vi "Aplicacion.vi"() -> ()   [LabVIEW 2016]
uses:
  <vilib>/addons/database/Connection.llb/Conn ObjectReference.ctl
  <vilib>/addons/database/Connection.llb/DB Tools Open Connec (Path).vi
  <vilib>/Instr/_visa.llb/VISA Configure Serial Port (Instr).vi
  <vilib>/addons/database/Connection.llb/Conn Execute.vi
  <vilib>/addons/database/Recordset.llb/Rec Destroy - Connection.vi
  <vilib>/Utility/config.llb/Read Key (String).vi
  <vilib>/Utility/config.llb/Write Key (String).vi
  <vilib>/addons/database/NI_Database_API.lvlib
  <vilib>/Utility/config.llb/NI_LVConfig.lvlib
panel:
  out "Ready":bool
  out "Condition":string
  out "Table":string
  in  "Read/Write Auto":bool
  out "retry":bool=TRUE
  out "Errores":errorcluster[](array[cluster])
  in  "Retry Conection":bool
  out "Errors":string[](array[string])
  in  "Configuration":bool caption="Blank Button"
  in  "Registers":bool caption="Blank Button"
  in  "Monitor":bool caption="Blank Button"
  in  "Tab Control":enum32{"Monitor", "Registers", "Configuration"}(tab)
  out "Graph":dbl(graph)
  in  "Conection Type":string(combo)="VISA"
  in  "To":timestamp
  in  "From":timestamp
  out "Data":i32(listbox)
  in  "Get Data":bool
  in  "Aply filter":bool
  in  "Section":string(combo)
  in  "Edit Config":bool
  in  "Data":string[][](table)
  in  "Save":bool
  in  "Delete Data":bool
  out "Modbus Request":string
  in  "Quantity":u8=1
  in  "Address":u8=1
  in  "Function Code":u8(ring)=1 items=["Read Coils"=1, "Read Discrete Inputs"=2, "Read Holding Registers"=3, "Read Input Register"=4, "Write Single Coil"=5, "Write Single Register"=6]
  out "Conections":T1
  out "Byte Count":i32 format="%02.0f"
  out "Function Code":i32 format="%02.0f"
  in  "Conection":string(combo)="VISA"
  in  "Read/Write Data":bool
  out "Modbus Response":string
  out "Data":dbl format="%#_4g"
  in  "parity (0:none)":enum16{"None", "Odd", "Even", "Mark", "Space"}(ring)
  in  "Cluster Conections":T1 {"VISAs"."Stop bit" items=["1.0"=10, "1.5"=15, "2.0"=20]; "VISAs"."Parity" items=["No parity", "Odd parity", "Even parity", "Mark parity", "Space parity"]}
  out "Final Error":errorcluster
  in  "stop":bool
  # "Universidad Autonoma de Queretaro"
  # "Facultad de Informatica"
  # "Desarrollo de Intefaces de Hardware II"
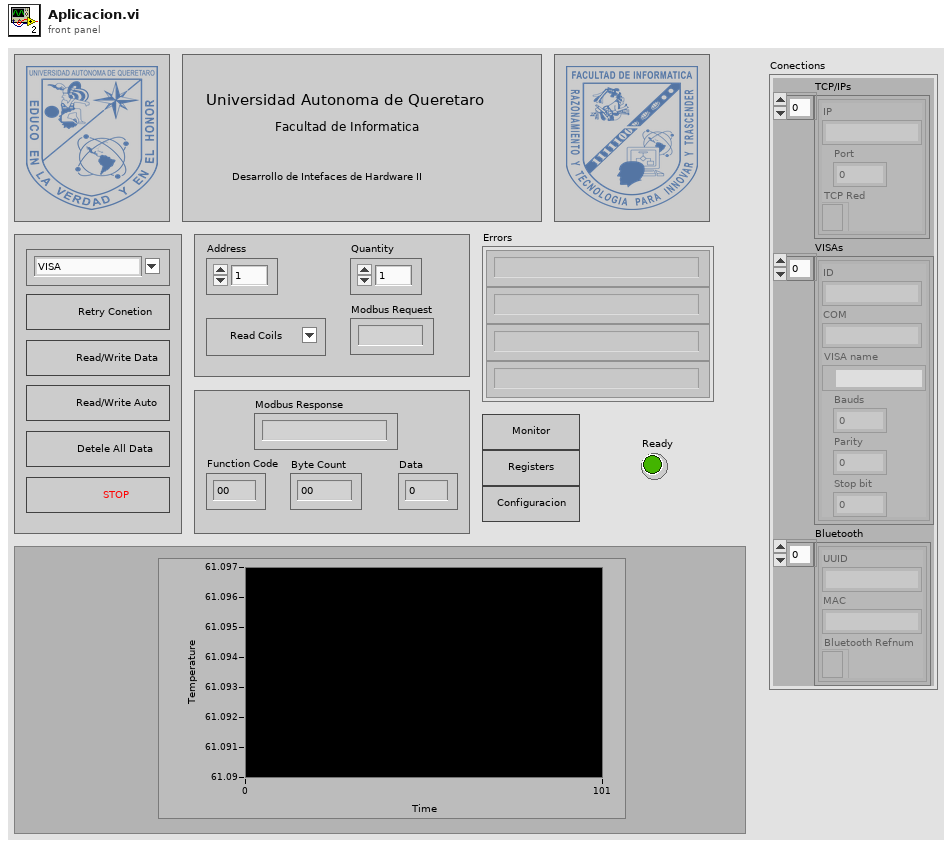
[diagram p1: front panel]
types:
  T1 = cluster{"TCP/IPs":cluster{"IP":string, "Port":u16, "TCP Red":refnum<k5>}[], "VISAs":cluster{"ID":string, "COM":string, "VISA name":refnum<visa-resource-name>, "Bauds":dbl, "Parity":u16, "Stop bit":u16}[], "Bluetooth":cluster{"UUID":string, "MAC":string, "Bluetooth Refnum":refnum<k31>}[]}
  T2 = enum16{"Standard", "Buffered", "CRLF", "Immediate"}
  T3 = enum8{"Enabled", "Disabled", "Disabled and Grayed Out"}
  T4 = typedef "NI_LVConfig.lvlib/Config Data RefNum.ctl" = refnum<k1>
  T5 = typedef "NI_Database_API.lvlib/Conn ObjectReference.ctl" = refnum<k1>
  T6 = cluster{"IP":string, "Port":u16, "TCP Red":refnum<k5>}[]
  T7 = cluster{"IP":string, "Port":u16, "TCP Red":refnum<k5>}
  T8 = cluster{"IP":string, "Port":u16, "connection ID":refnum<k5>}
  T9 = cluster{"IP":string, "Port":u16, "connection ID":refnum<k5>}[]
  T10 = cluster{"ID":string, "COM":string, "VISA name":refnum<visa-resource-name>, "Bauds":dbl, "Parity":u16, "Stop bit":u16}[]
  T11 = cluster{"ID":string, "COM":string, "VISA name":refnum<visa-resource-name>, "Bauds":dbl, "Parity":u16, "Stop bit":u16}
  T12 = cluster{"UUID":string, "MAC":string, "Bluetooth Refnum":refnum<k31>}[]
  T13 = cluster{"UUID":string, "MAC":string, "Bluetooth Refnum":refnum<k31>}
  T14 = cluster{"UUID":string, "UUID":string, "connection ID":refnum<k31>}
  T15 = cluster{"UUID":string, "UUID":string, "connection ID":refnum<k31>}[]
  T16 = typedef "NI_Database_API.lvlib/Rec ObjectReference.ctl" = refnum<k1>
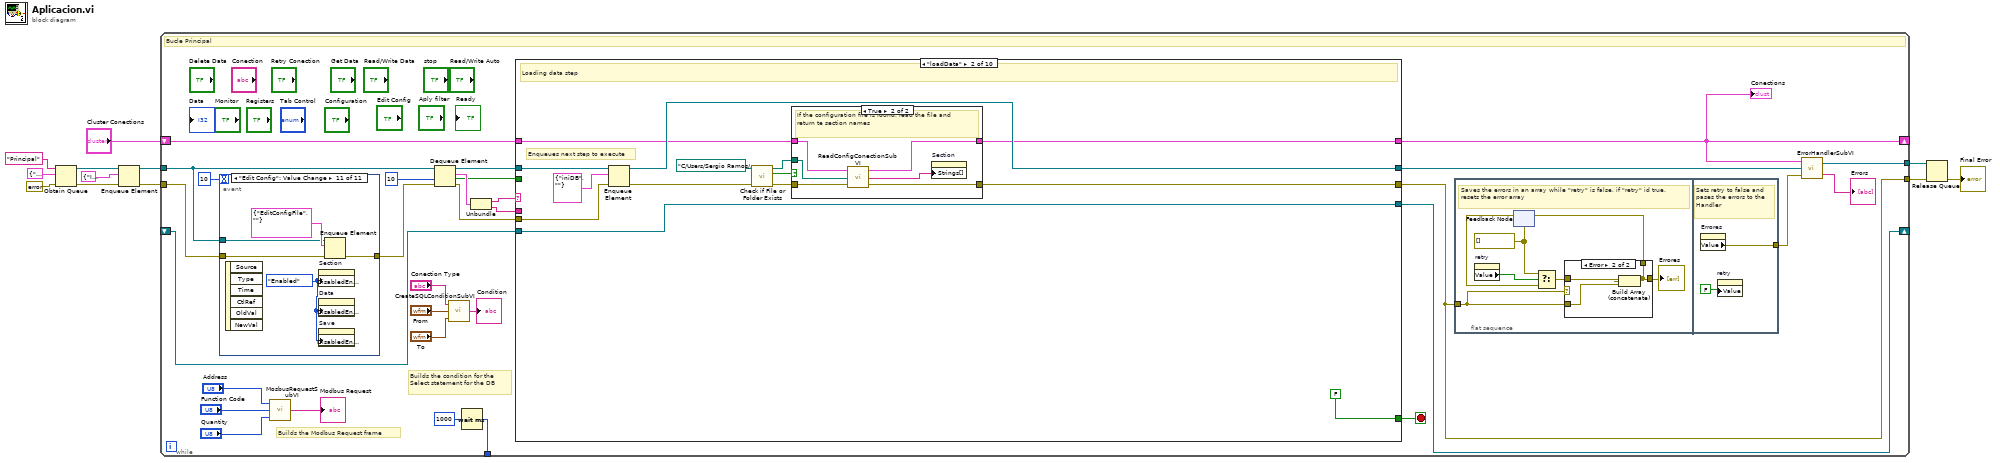
[diagram p0: block diagram]
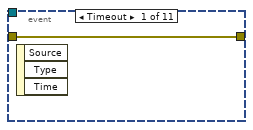
[diagram p3: hidden frame]
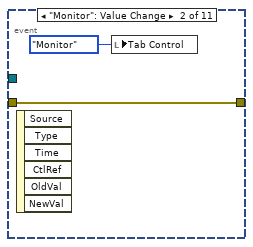
[diagram p4: hidden frame]
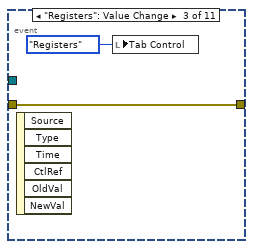
[diagram p5: hidden frame]
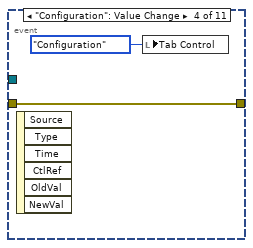
[diagram p6: hidden frame]
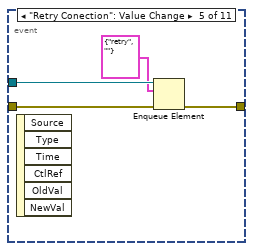
[diagram p7: hidden frame]
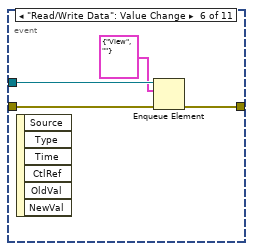
[diagram p8: hidden frame]
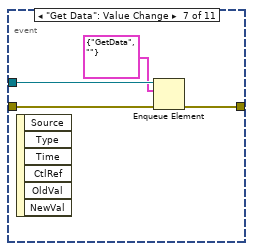
[diagram p9: hidden frame]
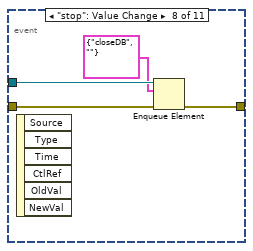
[diagram p10: hidden frame]
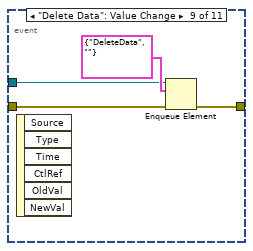
[diagram p11: hidden frame]
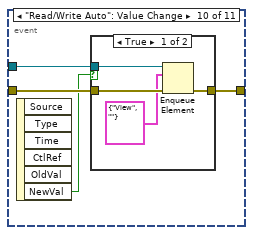
[diagram p12: hidden frame]
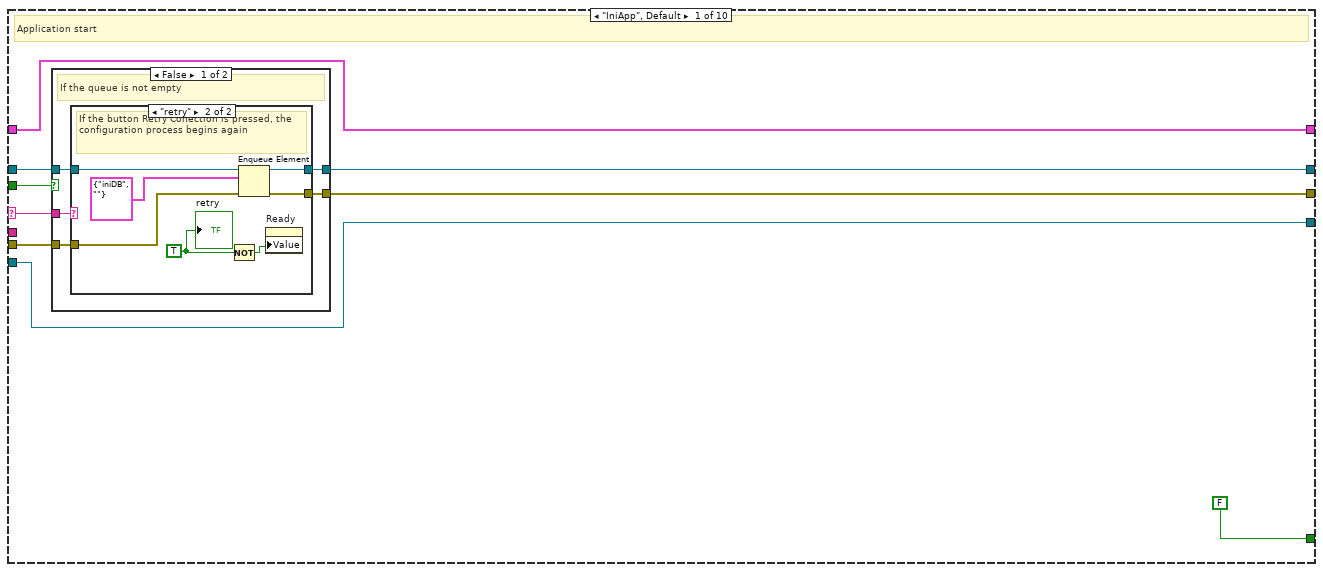
[diagram p14: hidden frame]
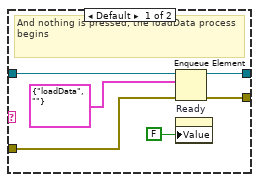
[diagram p15: hidden frame]
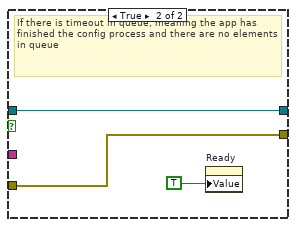
[diagram p16: hidden frame]
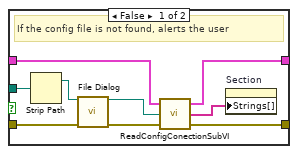
[diagram p17: hidden frame]
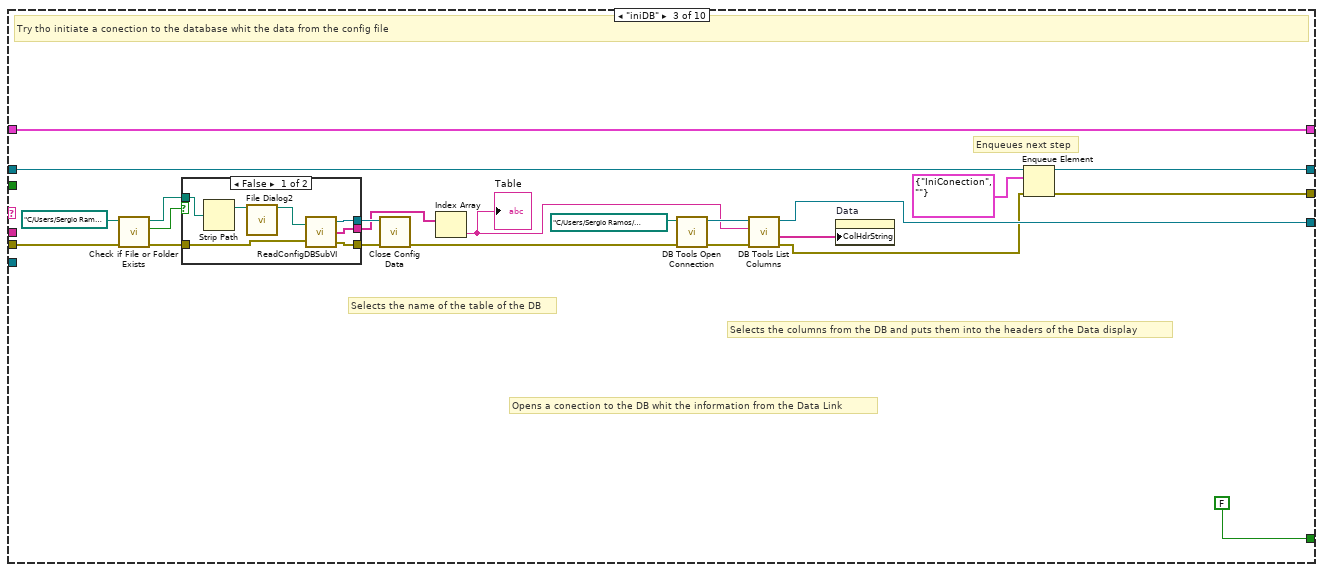
[diagram p18: hidden frame]
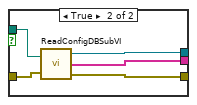
[diagram p19: hidden frame]
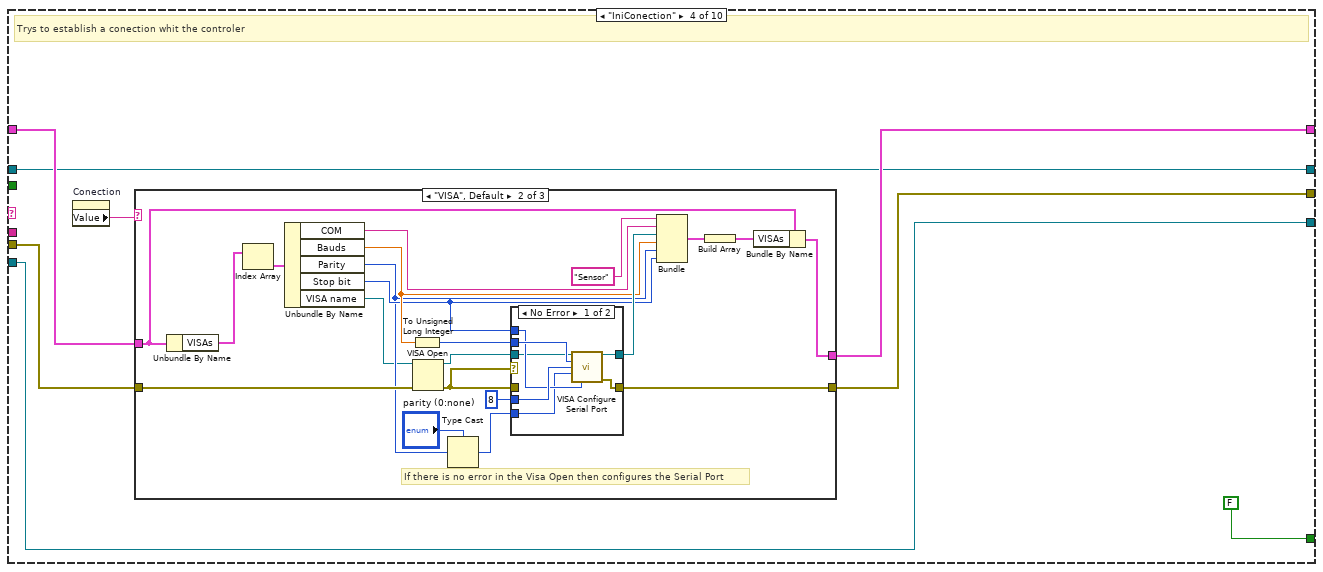
[diagram p20: hidden frame]
diagram:
  n1 = Obtain Queue(name (unnamed)="Principal", element data type=cluster{string, string} {"", ""}, error in (no error)=errorcluster {"status"=FALSE, "code"=0, "source"=""}) -> (queue out=w6:refnum<queue>, error out=w4:errorcluster)  [unwired: 2 in, 1 out]
  n2 = Enqueue Element(queue=w6, element=cluster{string, string} {"IniApp", ""}, error in (no error)=w4) -> (queue out=w5:refnum<queue>, error out=w3:errorcluster)  [unwired: 1 in, 1 out]
  n3 = while {
    tunnel: w5 -> [w30]
    shift-right: [w19] -> _
    shift-left: "Cluster Conections" -> [w41]
    shift-right: [w26] -> _
    shift-left: _ -> [w14]
    tunnel: [w29] -> _
    tunnel: w3 -> [w27]
    tunnel: [w23] -> w2
    tunnel: [w22] -> w1
    stop <- w20 stop-if-true
    # "Builds the Modbus Request frame"
    # "Builds the condition for the Select statement for the DB"
    # "Bucle Principal"
    n4 = event shown="[10] \"Edit Config\": Value Change" {
      selector: _ -> [_ _ _ _ _ _ _ _ _ _ _]
      dyn-events: _ -> [_ _ _ _ _ _ _ _ _ _ _]
      timeout: 10 -> [_ _ _ _ _ _ _ _ _ _ _]
      tunnel: w30 -> [_ _ _ _ w67 w71 w75 w79 w82 w87 w96]
      tunnel: w27 -> [w57 w58 w60 w62 w65 w69 w74 w77 w81 w86 w95]
      tunnel: [w57 w58 w60 w62 w64 w68 w73 w76 w80 w85 w94] -> w13
      event Timeout {
        n5 = event-data() -> ()  [unwired: 1 in, 3 out]
      }
      event "Monitor": Value Change {
        n6 = event-data() -> ()  [unwired: 1 in, 6 out]
        n7 = local write "Tab Control"(enum32{"Monitor", "Registers", "Configuration"}."Monitor" ("Tab Control")) -> ()
      }
      event "Registers": Value Change {
        n8 = event-data() -> ()  [unwired: 1 in, 6 out]
        n9 = local write "Tab Control"(enum32{"Monitor", "Registers", "Configuration"}."Registers" ("Tab Control")) -> ()
      }
      event "Configuration": Value Change {
        n10 = event-data() -> ()  [unwired: 1 in, 6 out]
        n11 = local write "Tab Control"(enum32{"Monitor", "Registers", "Configuration"}."Configuration" ("Tab Control")) -> ()
      }
      event "Retry Conection": Value Change {
        n12 = event-data() -> ()  [unwired: 1 in, 6 out]
        n13 = Enqueue Element(queue=w67, element=cluster{string, string} {"retry", ""}, error in (no error)=w65) -> (error out=w64:errorcluster)  [unwired: 1 in, 2 out]
      }
      event "Read/Write Data": Value Change {
        n14 = event-data() -> ()  [unwired: 1 in, 6 out]
        n15 = Enqueue Element(queue=w71, element=cluster{string, string} {"View", ""}, error in (no error)=w69) -> (error out=w68:errorcluster)  [unwired: 1 in, 2 out]
      }
      event "Get Data": Value Change {
        n16 = event-data() -> ()  [unwired: 1 in, 6 out]
        n17 = Enqueue Element(queue=w75, element=cluster{string, string} {"GetData", ""}, error in (no error)=w74) -> (error out=w73:errorcluster)  [unwired: 1 in, 2 out]
      }
      event "stop": Value Change {
        n18 = event-data() -> ()  [unwired: 1 in, 6 out]
        n19 = Enqueue Element(queue=w79, element=cluster{string, string} {"closeDB", ""}, error in (no error)=w77) -> (error out=w76:errorcluster)  [unwired: 1 in, 2 out]
      }
      event "Delete Data": Value Change {
        n20 = event-data() -> ()  [unwired: 1 in, 6 out]
        n21 = Enqueue Element(queue=w82, element=cluster{string, string} {"DeleteData", ""}, error in (no error)=w81) -> (error out=w80:errorcluster)  [unwired: 1 in, 2 out]
      }
      event "Read/Write Auto": Value Change {
        n22 = event-data() -> ("NewVal"=w84:bool)  [unwired: 1 in, 5 out]
        n23 = case shown="True" w84 {
          tunnel: w87 -> [w91 _]
          tunnel: w86 -> [w90 w92]
          tunnel: [w88 w92] -> w85
          frame True {
            n24 = Enqueue Element(queue=w91, element=cluster{string, string} {"View", ""}, error in (no error)=w90) -> (error out=w88:errorcluster)  [unwired: 1 in, 2 out]
          }
          frame False {
          }
        }
      }
      event "Edit Config": Value Change {
        w93 = T3."Enabled" ("Disabled")
        n25 = event-data() -> ()  [unwired: 1 in, 6 out]
        n26 = property on="Section" class="CmbBox"("DisabledEnum"=w93) -> ()  [unwired: 2 in, 2 out]
        n27 = property on="Data" class="Tbl (strict)"("DisabledEnum"=w93) -> ()  [unwired: 2 in, 2 out]
        n28 = property on="Save" class="Bool"("DisabledEnum"=w93) -> ()  [unwired: 2 in, 2 out]
        n29 = Enqueue Element(queue=w96, element=cluster{string, string} {"EditConfigFile", ""}, error in (no error)=w95) -> (error out=w94:errorcluster)  [unwired: 1 in, 2 out]
      }
    }
    n30 = call "MosbusRequestSubVI.vi"("Quantity"="Quantity", "Function Code"="Function Code", "Address"="Address") -> ("Modbus Request"=→"Modbus Request":string)
    n31 = Dequeue Element(queue=w30, timeout in ms (-1)=10, error in (no error)=w13) -> (queue out=w40:refnum<queue>, element=w43:cluster{string, string}, timed out?=w35:bool, error out=w39:errorcluster)
    n32 = call "CreateSQLConditionSubVI.vi"("To"="To", "From"="From", "Conection Type"="Conection Type") -> ("Condition"=→"Condition":string)
    n33 = Wait (ms)(milliseconds to wait=u32 1000) -> (millisecond timer value=w29:u32)
    n34 = Unbundle(w43) -> (w42:string, w38:string)
    n35 = case shown="\"loadData\"" w42 {
      selector: w42 -> [w100 _ _ _ _ _ _ _ w411 _]
      tunnel: w41 -> [w98 w138 w174 w195 w258 w300 w325 w403 w412 w462]
      tunnel: [w98 w137 w174 w198 w258 w300 w318 w403 w413 w462] -> w19
      tunnel: w40 -> [w105 w140 w164 w193 w259 w297 w323 w401 w414 w461]
      tunnel: w39 -> [w106 w141 w166 w194 w272 w307 w316 w399 w410 w457]
      tunnel: [w104 w139 w163 w193 w259 w296 w321 w400 w414 w461] -> w24
      tunnel: w38 -> [_ _ _ _ _ _ w324 _ _ _]
      tunnel: [w103 w129 w160 w196 w253 w301 w319 w405 w408 w453] -> w26
      tunnel: w14 -> [w103 w129 _ w196 w260 w306 w320 w404 w408 w453]
      tunnel: [w102 w131 w158 w191 w257 w295 w322 w398 w409 w454] -> w23
      tunnel: w35 -> [w101 _ _ _ _ _ _ _ _ _]
      tunnel: [FALSE FALSE FALSE FALSE FALSE FALSE FALSE FALSE TRUE FALSE] -> w20
      frame "IniApp", Default {
        # "Application start"
        n36 = case shown="False" w101 {
          tunnel: w106 -> [w111 w126]
          tunnel: w105 -> [w110 w127]
          tunnel: [w109 w127] -> w104
          tunnel: [w108 w126] -> w102
          tunnel: w100 -> [w107 _]
          frame False {
            # "If the queue is not empty"
            n37 = case shown="\"retry\"" w107 {
              tunnel: w111 -> [w117 w120]
              tunnel: w110 -> [w116 w121]
              tunnel: [w115 w124] -> w109
              tunnel: [w113 w122] -> w108
              frame Default {
                # "And nothing is pressed, the loadData process begins"
                n38 = Enqueue Element(queue=w116, element=cluster{string, string} {"loadData", ""}, error in (no error)=w117) -> (queue out=w115:refnum<queue>, error out=w113:errorcluster)  [unwired: 1 in, 1 out]
                n39 = property on="Ready" class="Bool (strict)"("Value"=FALSE) -> ()  [unwired: 2 in, 2 out]
              }
              frame "retry" {
                w119 = TRUE
                # "If the button Retry Conection is pressed, the configuration process begins again"
                n40 = Not(x=w119) -> (.not. x?=w118:bool)
                n41 = Enqueue Element(queue=w121, element=cluster{string, string} {"iniDB", ""}, error in (no error)=w120) -> (queue out=w124:refnum<queue>, error out=w122:errorcluster)  [unwired: 1 in, 1 out]
                n42 = property on="Ready" class="Bool (strict)"("Value"=w118) -> ()  [unwired: 2 in, 2 out]
                "retry" <- w119
              }
            }
          }
          frame True {
            # "If there is timeout in queue, meaning the app has finished the config process and there are no elements in queue"
            n43 = property on="Ready" class="Bool (strict)"("Value"=TRUE) -> ()  [unwired: 2 in, 2 out]
          }
        }
      }
      frame "loadData" {
        # "Enqueues next step to execute"
        # "Loading data step"
        n44 = Enqueue Element(queue=w140, element=cluster{string, string} {"iniDB", ""}, error in (no error)=w141) -> (queue out=w139:refnum<queue>, error out=w132:errorcluster)  [unwired: 1 in, 1 out]
        n45 = call <vilib>:"Check if File or Folder Exists.vi"("error in (no error)"=w132, "path"=path "C:/Users/Sergio Ramos/Documents/UAQ/Desarrollo de Interfaces de Hardware II/Proyecto-DIHII/Configuraciones/config2.ini" ("file path (use dialog)")) -> ("error out"=w136:errorcluster, "file or folder exists?"=w133:bool, "dup path"=w134:path)  [unwired: 7 in]
        n46 = case shown="True" w133 {
          tunnel: [w147 w156] -> w131
          tunnel: w138 -> [w145 w154]
          tunnel: [w146 w155] -> w137
          tunnel: w136 -> [w148 w152]
          tunnel: w134 -> [w149 w153]
          frame False {
            # "If the config file is not found, alerts the user"
            n47 = Strip Path(path=w149) -> (stripped path=w150:path)  [unwired: 1 out]
            n48 = call "File Dialog"("start path"=w150, "error in"=w148) -> ("selected path"=w144:path, "error out"=w143:errorcluster)  [unwired: 10 in, 2 out]
            n49 = call "ReadConfigConectionSubVI.vi"("error in (no error)"=w143, "dup path"=w144, "Conections in"=w145) -> ("error out"=w147:errorcluster, "section names"=w142:string[], "Conections out"=w146:T1)
            n50 = property on="Section" class="CmbBox"("Strings[]"=w142) -> ()  [unwired: 2 in, 2 out]
          }
          frame True {
            # "If the configuration file is found, read the file and return te section names"
            n51 = call "ReadConfigConectionSubVI.vi"("error in (no error)"=w152, "dup path"=w153, "Conections in"=w154) -> ("error out"=w156:errorcluster, "section names"=w151:string[], "Conections out"=w155:T1)
            n52 = property on="Section" class="CmbBox"("Strings[]"=w151) -> ()  [unwired: 2 in, 2 out]
          }
        }
      }
      frame "iniDB" {
        # "Enqueues next step"
        # "Selects the columns from the DB and puts them into the headers of the Data display"
        # "Opens a conection to the DB whit the information from the Data Link"
        # "Selects the name of the table of the DB"
        # "Try tho initiate a conection to the database whit the data from the config file"
        n53 = call <vilib>:"Check if File or Folder Exists.vi"("error in (no error)"=w166, "path"=path "C:/Users/Sergio Ramos/Documents/UAQ/Desarrollo de Interfaces de Hardware II/Proyecto-DIHII/Configuraciones/config2.ini" ("file path (use dialog)")) -> ("error out"=w171:errorcluster, "file or folder exists?"=w167:bool, "dup path"=w172:path)  [unwired: 7 in]
        n54 = case shown="False" w167 {
          tunnel: w172 -> [w185 w189]
          tunnel: w171 -> [w183 w190]
          tunnel: [w179 w187] -> w170
          tunnel: [w181 w186] -> w169
          tunnel: [w180 w188] -> w157
          frame False {
            n55 = Strip Path(path=w185) -> (stripped path=w184:path)  [unwired: 1 out]
            n56 = call "File Dialog2"("start path"=w184) -> ("selected path"=w182:path)  [unwired: 11 in, 3 out]
            n57 = call "ReadConfigDBSubVI.vi"("DB File Path"=w182, "error in (no error)"=w183) -> ("Refnum out"=w181:T4, "DB Elements"=w180:string[], "error out"=w179:errorcluster)
          }
          frame True {
            n58 = call "ReadConfigDBSubVI.vi"("DB File Path"=w189, "error in (no error)"=w190) -> ("Refnum out"=w186:T4, "DB Elements"=w188:string[], "error out"=w187:errorcluster)
          }
        }
        n59 = call <vilib>:"Close Config Data.vi"("error in (no error)"=w170, "refnum"=w169) -> ("error out"=w168:errorcluster)  [unwired: 8 in, 1 out]
        n60 = Index Array(array=w157) -> (element=w161:string)  [unwired: 1 in]
        "Table" <- w161
        n61 = call-poly <vilib>:"DB Tools Open Connection.vi"("error in (no error)"=w168, "connection information"=path "C:/Users/Sergio Ramos/Documents/UAQ/Desarrollo de Interfaces de Hardware II/Proyecto-DIHII/SQLServerDB.udl") -> ("error out"=w177:errorcluster, "connection reference"=w176:T5)  [unwired: 6 in]
        n62 = call <vilib>:"DB Tools List Columns.vi"("error in (no error)"=w177, "table"=w161, "connection reference"=w176) -> ("error out"=w159:errorcluster, "columns"=w178:string[], "connection reference out"=w160:T5)  [unwired: 1 in, 1 out]
        n63 = property on="Data" class="MCListbox (strict)"("ColHdrString"=w178) -> ()  [unwired: 2 in, 2 out]
        n64 = Enqueue Element(queue=w164, element=cluster{string, string} {"IniConection", ""}, error in (no error)=w159) -> (queue out=w163:refnum<queue>, error out=w158:errorcluster)  [unwired: 1 in, 1 out]
      }
      frame "IniConection" {
        # "Trys to establish a conection whit the controler"
        n65 = property on="Conection" class="CmbBox"() -> ("Value"=w197:string)  [unwired: 2 in, 2 out]
        n66 = case shown="\"VISA\", Default" w197 {
          tunnel: [w209 w227 w248] -> w191
          tunnel: w195 -> [w201 w230 w243]
          tunnel: [w207 w229 w242] -> w198
          tunnel: w194 -> [w199 w228 w247]
          frame "TCP" {
            n67 = Unbundle By Name(w201) -> ("TCP/IPs"=w200:T6)
            n68 = Index Array(array=w200) -> (element=w208:T7)  [unwired: 1 in]
            n69 = Unbundle By Name(w208) -> ("IP"=w206:string, "Port"=w205:u16)
            n70 = TCP Open Connection(address=w206, remote port or service name=w205, error in (no error)=w199) -> (connection ID=w204:refnum<k5>, error out=w209:errorcluster)  [unwired: 2 in]
            n71 = Bundle("IP"=w206, "Port"=w205, "connection ID"=w204) -> (w203:T8)  [unwired: 1 in]
            n72 = Build Array(w203) -> (w202:T9)
            n73 = Bundle By Name(cluster=w201, "TCP/IPs"=w202) -> (w207:T1)
          }
          frame "VISA", Default {
            # "If there is no error in the Visa Open then configures the Serial Port"
            n74 = Unbundle By Name(w230) -> ("VISAs"=w225:T10)
            n75 = Index Array(array=w225) -> (element=w224:T11)  [unwired: 1 in]
            n76 = Unbundle By Name(w224) -> ("COM"=w219:string, "Bauds"=w217:dbl, "Parity"=w213:u16, "Stop bit"=w216:u16, "VISA name"=w210:refnum<visa-resource-name>)
            n77 = To Unsigned Long Integer(number=w217) -> (unsigned 32bit integer=w223:u32)
            n78 = VISA Open(error in (no error)=w228, VISA resource name=w210) -> (VISA resource name=w211:refnum<visa-resource-name>, error out=w226:errorcluster)  [unwired: 3 in]
            n79 = Type Cast(type="parity (0:none)", x=w213) -> (*(type *) &x=w212:enum16{"None", "Odd", "Even", "Mark", "Space"})
            n80 = case shown="No Error" w226 {
              tunnel: [w237 w238] -> w227
              tunnel: w223 -> [w236 _]
              tunnel: u16 8 ("data bits (8)") -> [w235 _]
              tunnel: [w234 w239] -> w218
              tunnel: w216 -> [w233 _]
              tunnel: w212 -> [w232 _]
              tunnel: w211 -> [w231 w239]
              tunnel: w226 -> [_ w238]
              frame No Error {
                n81 = call-poly "VISA Configure Serial Port"("VISA resource name"=w231, "baud rate (9600)"=w236, "data bits (8)"=w235, "parity (0:none)"=w232, "stop bits (10: 1 bit)"=w233) -> ("VISA resource name out"=w234:refnum<visa-resource-name>, "error out"=w237:errorcluster)  [unwired: 9 in]
              }
              frame Error {
              }
            }
            n82 = Bundle("ID"="Sensor", "COM"=w219, "VISA name"=w218, "Bauds"=w217, "Parity"=w213, "Stop bit"=w216) -> (w215:T11)  [unwired: 1 in]
            n83 = Build Array(w215) -> (w214:T10)
            n84 = Bundle By Name(cluster=w230, "VISAs"=w214) -> (w229:T1)
          }
          frame "Bluetooth" {
            n85 = Unbundle By Name(w243) -> ("Bluetooth"=w250:T12)
            n86 = Index Array(array=w250) -> (element=w249:T13)  [unwired: 1 in]
            n87 = Unbundle By Name(w249) -> ("UUID"=w245:string, "MAC"=w241:string)
            n88 = Bluetooth Open Connection(6:w245, 8:w247, 11:w241) -> (0:w248:errorcluster, 3:w246:refnum<k31>)  [unwired: 2 in]
            n89 = Bundle("UUID"=w245, "UUID"=w245, "connection ID"=w246) -> (w244:T14)  [unwired: 1 in]
            n90 = Build Array(w244) -> (w240:T15)
            n91 = Bundle By Name(cluster=w243, "Bluetooth"=w240) -> (w242:T1)
          }
        }
      }
      frame "GetData" {
        # "Configures the Data table to diplay all the elements"
        # "Displays the data in the table"
        # "Converts the returned data to an array of strings"
        # "If the Aply filter is activated, adds the condition to the Select Data controls"
        # "Reads the data from the DB and displays it"
        n92 = property on="Aply filter" class="Bool (strict)"() -> ("Value"=w251:bool)  [unwired: 2 in, 2 out]
        n93 = case shown="True" w251 {
          tunnel: ["" ("Value") w274] -> w252
          frame False {
          }
          frame True {
            n94 = property on="Condition" class="Str"() -> ("Value"=w274:string)  [unwired: 2 in, 2 out]
          }
        }
        n95 = property on="Table" class="Str"() -> ("Value"=w254:string)  [unwired: 2 in, 2 out]
        n96 = call <vilib>:"DB Tools Select Data.vi"("condition"=w252, "error in (no error)"=w272, "columns"=string[] ["ID", "Fecha", "Hora", "Tipo", "Temperatura", "SensorX", "SensorY", "SensorZ", "TCP"], "table"=w254, "connection reference"=w260) -> ("error out"=w267:errorcluster, "data"=w269:variant[][], "connection reference out"=w253:T5)  [unwired: 1 in]
        n97 = Variant To Data(error in=w267, type=string[][] [], Variant=w269) -> (data=w256:string[][], error out=w257:errorcluster)
        n98 = Index Array(array=w256) -> (element=w266:string[])  [unwired: 2 in]
        n99 = Array Size(array=w256) -> (size(s)=w265:i32[])
        n100 = property on="Data" class="MCListbox (strict)"("ItemNames"=w256) -> ()  [unwired: 2 in, 2 out]
        n101 = Index Array(array=w265) -> (element=w264:i32)  [unwired: 1 in]
        n102 = Array Size(array=w266) -> (size(s)=w262:i32)
        n103 = Increment(x=w264) -> (x+1=w263:i32)
        n104 = flat-sequence {
          tunnel: w262 -> [w276]
          tunnel: [w276] -> w271
          tunnel: w263 -> [w275]
          tunnel: [w275] -> w270
          tunnel: w271 -> [w288]
          tunnel: w270 -> [w285]
          frame #0 {
            # "Sets a width to eash ActiveCell"
            n105 = for {
              N: w276 -> [_]
              tunnel: w275 -> [w277]
              i -> [w278]
              n106 = for {
                N: w277 -> [_]
                tunnel: w278 -> [w283]
                i -> [w282]
                n107 = Bundle(w282, w283) -> (w281:cluster{i32, i32})  [unwired: 1 in]
                n108 = property on="Data" class="MCListbox (strict)"("Width"=u32 75 ("Active Cell:Cell Size:Width"), "Justify"=enum16{"Left", "Center", "Right"}."Center" ("Active Cell:Cell Justification")) -> ()  [unwired: 2 in, 2 out]
                n109 = property on="Data" class="MCListbox (strict)"("ActiveCell"=w281) -> ()  [unwired: 2 in, 2 out]
              }
            }
          }
          frame #1 {
            w284 = u32 8 ("y")
            # "Sets the number of rows to diplay and if the ScrollBar is visible or not"
            n110 = Decrement(x=w285) -> (x-1=w286:i32)
            n111 = property on="Data" class="MCListbox (strict)"("NumCols"=w288) -> ()  [unwired: 2 in, 2 out]
            n112 = Greater Or Equal?(x=w286, y=w284) -> (x >= y?=w287:bool)
            n113 = case shown="False" w287 {
              selector: w287 -> [w289 w291]
              tunnel: w286 -> [w290 _]
              tunnel: w284 -> [_ w292]
              frame False {
                n114 = property on="Data" class="MCListbox (strict)"("VScrollVis"=w289, "NumRows"=w290) -> ()  [unwired: 2 in, 2 out]
              }
              frame True {
                n115 = property on="Data" class="MCListbox (strict)"("VScrollVis"=w291, "NumRows"=w292) -> ()  [unwired: 2 in, 2 out]
              }
            }
          }
        }
      }
      frame "DeleteData" {
        # "If there is no error enqueues next step"
        # "Resets the ID of the table for the next inputs"
        # "Deletes all the data from the DB"
        n116 = property on="Table" class="Str"() -> ("Value"=w293:string)  [unwired: 2 in, 2 out]
        n117 = call <vilib>:"DB Tools Delete Data.vi"("condition"="", "error in (no error)"=w307, "table"=w293, "connection reference"=w306) -> ("error out"=w305:errorcluster, "connection reference out"=w298:T5)  [unwired: 6 in]
        n118 = call-poly <vilib>:"DB Tools Execute Query.vi"("error in (no error)"=w305, "SQL query"="DBCC CHECKIDENT ('elementos', RESEED, 0);", "connection reference"=w298) -> ("error out"=w303:errorcluster, "recordset reference"=w302:T16)  [unwired: 5 in]
        n119 = call-poly <vilib>:"DB Tools Free Object.vi"("error in (no error)"=w303, "recordset reference"=w302) -> ("error out"=w308:errorcluster, "connection reference"=w301:T5)  [unwired: 8 in]
        n120 = case shown="No Error" w308 {
          tunnel: w297 -> [w313 w314]
          tunnel: [w312 w314] -> w296
          tunnel: [w310 w315] -> w295
          tunnel: w308 -> [w309 w315]
          frame No Error {
            n121 = Enqueue Element(queue=w313, element=cluster{string, string} {"GetData", ""}, error in (no error)=w309) -> (queue out=w312:refnum<queue>, error out=w310:errorcluster)  [unwired: 1 in, 1 out]
          }
          frame Error {
          }
        }
      }
      frame "View" {
        # "Writes and reads from the controler, and insert the data into the DB"
        n122 = while {
          tunnel: w324 -> [w335]
          tunnel: w320 -> [w330]
          tunnel: [w329] -> w319
          tunnel: w323 -> [w334]
          tunnel: [w332] -> w321
          tunnel: w316 -> [w331]
          tunnel: [w333] -> w322
          tunnel: w325 -> [w336]
          tunnel: [w328] -> w318
          stop <- w326 stop-if-true
          n123 = case shown="\"VISA\", Default" w335 {
            tunnel: [w342 w385] -> w333
            tunnel: w336 -> [w358 w384]
            tunnel: [w358 w384] -> w328
            tunnel: w334 -> [w349 w383]
            tunnel: [w348 w383] -> w332
            tunnel: w331 -> [w352 w387]
            tunnel: w330 -> [w353 w382]
            tunnel: [w338 w382] -> w329
            frame "VISA", Default {
              # "Reads the response from the controler"
              # "Select the VISA resource name from the conections and writes the Modbus Request"
              n124 = Unbundle By Name(w358) -> ("VISAs"=w357:T10)
              n125 = Index Array(array=w357) -> (element=w356:T11)  [unwired: 1 in]
              n126 = property on="Modbus Request" class="Str"() -> ("Value"=w347:string)  [unwired: 2 in, 2 out]
              n127 = Unbundle By Name(w356) -> ("VISA name"=w341:refnum<visa-resource-name>)
              n128 = VISA Write(VISA resource name=w341, write buffer=w347, error in (no error)=w352) -> (VISA resource name out=w355:refnum<visa-resource-name>, error out=w339:errorcluster)  [unwired: 1 out]
              n129 = VISA Read(VISA resource name=w355, byte count=u32 20, error in (no error)=w339) -> (read buffer=w346:string, error out=w354:errorcluster)  [unwired: 2 out]
              "Modbus Response" <- w346
              n130 = call "MosbusResponseSubVI.vi"("read buffer"=w346) -> ("Function Code"=→"Function Code":i32, "Byte Count"=→"Byte Count":i32, "Data"=w345:dbl)
              "Graph" <- w345
              n131 = flat-sequence {
                tunnel: w353 -> [w366]
                tunnel: w354 -> [w367]
                tunnel: [w367] -> w351
                tunnel: [w366] -> w350
                tunnel: w345 -> [w365]
                tunnel: [w371] -> w337
                tunnel: [w370] -> w338
                tunnel: w351 -> [w369]
                tunnel: w350 -> [w368]
                frame #0 {
                  "Data" <- w365
                }
                frame #1 {
                  n132 = case shown="No Error" w369 {
                    tunnel: [w378 w380] -> w371
                    tunnel: [w377 w379] -> w370
                    tunnel: w368 -> [w374 w379]
                    tunnel: w369 -> [w373 w380]
                    frame No Error {
                      # "If there is no error in the Read/Write, inserts data into the DB"
                      n133 = property on="Data" class="DigNum (strict)"() -> ("Value"=w375:dbl)  [unwired: 2 in, 2 out]
                      n134 = property on="Conection" class="CmbBox"() -> ("Value"=w376:string)  [unwired: 2 in, 2 out]
                      n135 = property on="Table" class="Str"() -> ("Value"=w372:string)  [unwired: 2 in, 2 out]
                      n136 = call "InsertIntoDBSubVI.vi"("error in (no error)"=w373, "Conexion"=w376, "Tabla"=w372, "Refnum in"=w374, "Data"=w375) -> ("error out"=w378:errorcluster, "Refnum out"=w377:T5)
                    }
                    frame Error {
                    }
                  }
                }
              }
              n137 = case shown="No Error" w337 {
                tunnel: w349 -> [w362 w363]
                tunnel: [w361 w363] -> w348
                tunnel: [w359 w364] -> w342
                tunnel: w337 -> [_ w364]
                frame No Error {
                  # "Enqueues next step"
                  n138 = Enqueue Element(queue=w362, element=cluster{string, string} {"GetData", ""}) -> (queue out=w361:refnum<queue>, error out=w359:errorcluster)  [unwired: 2 in, 1 out]
                }
                frame Error {
                }
              }
            }
            frame "TCP" {
              n139 = Unbundle By Name(w384) -> ("TCP/IPs"=w389:T6)
              n140 = Index Array(array=w389) -> (element=w390:T7)  [unwired: 1 in]
              n141 = Unbundle By Name(w390) -> ("TCP Red"=w381:refnum<k5>)
              n142 = TCP Read(connection ID=w381, bytes to read=1500, error in (no error)=w387, 7:T2."Standard" ("mode (standard)")) -> (data out=w396:string, error out=w385:errorcluster)  [unwired: 1 in, 1 out]
              n143 = Match Pattern(string=w396, regular expression=":") -> (after substring=w394:string)  [unwired: 1 in, 3 out]
              n144 = Match Pattern(string=w394, regular expression=";") -> (before substring=w392:string)  [unwired: 1 in, 3 out]
              n145 = Decimal String To Number(string=w392) -> (number=w391:i32)  [unwired: 2 in, 1 out]
              n146 = To Double Precision Float(number=w391) -> ()  [unwired: 1 out]
            }
          }
          n147 = property on="Read/Write Auto" class="Bool (strict)"() -> ("Value"=w327:bool)  [unwired: 2 in, 2 out]
          n148 = Not(x=w327) -> (.not. x?=w326:bool)
        }
      }
      frame "closeDB" {
        w405 = T5 refnum items=["Connection"] ("connection reference out")
        # "Enqueues next step"
        # "Closes the conection with the DB"
        n149 = Enqueue Element(queue=w401, element=cluster{string, string} {"closeConection", ""}, error in (no error)=w399) -> (queue out=w400:refnum<queue>, error out=w406:errorcluster)  [unwired: 1 in, 1 out]
        n150 = call <vilib>:"DB Tools Close Connection.vi"("error in (no error)"=w406, "connection reference"=w404) -> ("error out"=w398:errorcluster)  [unwired: 5 in]
      }
      frame "closeConection" {
        # "Closes conection whit the controler"
        n151 = case shown="\"VISA\", Default" w411 {
          tunnel: [w416 w433 w443] -> w413
          tunnel: w412 -> [w418 w431 w445]
          tunnel: w410 -> [w426 w430 w442]
          tunnel: [w415 w429 w441] -> w409
          frame "VISA", Default {
            n152 = Unbundle By Name(w418) -> ("VISAs"=w428:T10)
            n153 = Index Array(array=w428) -> (element=w427:T11)  [unwired: 1 in]
            n154 = Unbundle By Name(w427) -> ("ID"=w423:string, "COM"=w424:string, "VISA name"=w425:refnum<visa-resource-name>, "Bauds"=w422:dbl, "Parity"=w421:u16, "Stop bit"=w420:u16)
            n155 = VISA Close(VISA resource name=w425, error in (no error)=w426) -> (error out=w415:errorcluster)
            n156 = Bundle("ID"=w423, "COM"=w424, "VISA name"=w425, "Bauds"=w422, "Parity"=w421, "Stop bit"=w420) -> (w419:T11)  [unwired: 1 in]
            n157 = Build Array(w419) -> (w417:T10)
            n158 = Bundle By Name(cluster=w418, "VISAs"=w417) -> (w416:T1)
          }
          frame "TCP" {
            n159 = Unbundle By Name(w431) -> ("TCP/IPs"=w440:T6)
            n160 = Index Array(array=w440) -> (element=w439:T7)  [unwired: 1 in]
            n161 = Unbundle By Name(w439) -> ("IP"=w434:string, "Port"=w435:u16, "TCP Red"=w438:refnum<k5>)
            n162 = TCP Close Connection(connection ID=w438, error in (no error)=w430) -> (connection ID out=w432:refnum<k5>, error out=w429:errorcluster)  [unwired: 1 in]
            n163 = Bundle("IP"=w434, "Port"=w435, "TCP Red"=w432) -> (w436:T7)  [unwired: 1 in]
            n164 = Build Array(w436) -> (w437:T6)
            n165 = Bundle By Name(cluster=w431, "TCP/IPs"=w437) -> (w433:T1)
          }
          frame "Bluetooth" {
            n166 = Unbundle By Name(w445) -> ("Bluetooth"=w452:T12)
            n167 = Index Array(array=w452) -> (element=w451:T13)  [unwired: 1 in]
            n168 = Unbundle By Name(w451) -> ("UUID"=w447:string, "MAC"=w448:string, "Bluetooth Refnum"=w450:refnum<k31>)
            n169 = TCP Close Connection(connection ID=w450, error in (no error)=w442) -> (connection ID out=w449:refnum<k31>, error out=w441:errorcluster)  [unwired: 1 in]
            n170 = Bundle("UUID"=w447, "MAC"=w448, "Bluetooth Refnum"=w449) -> (w446:T13)  [unwired: 1 in]
            n171 = Build Array(w446) -> (w444:T12)
            n172 = Bundle By Name(cluster=w445, "Bluetooth"=w444) -> (w443:T1)
          }
        }
      }
      frame "EditConfigFile" {
        # "Edits the values of the config file, allows to change one key each time"
        n173 = flat-sequence {
          tunnel: w457 -> [w465]
          tunnel: [w464] -> w456
          tunnel: [w463] -> w455
          tunnel: [w470] -> w459
          tunnel: [w469] -> w458
          tunnel: w456 -> [w468]
          tunnel: w455 -> [w467]
          tunnel: w459 -> [w503]
          tunnel: w458 -> [w500]
          tunnel: [w498] -> w454
          frame #0 {
            # "Opens config file to edit"
            n174 = call <vilib>:"Open Config Data.vi"("error in (no error)"=w465, "configuration file path"=path "C:/Users/Sergio Ramos/Documents/UAQ/Desarrollo de Interfaces de Hardware II/Proyecto-DIHII/Configuraciones/config2.ini" ("file path (use dialog)")) -> ("error out"=w464:errorcluster, "refnum"=w463:T4)  [unwired: 7 in, 1 out]
          }
          frame #1 {
            # "While the Save botton is not pressed, reads the values of the key selected"
            n175 = while {
              tunnel: w467 -> [w479]
              tunnel: w468 -> [w478]
              tunnel: [w473] -> w470
              tunnel: [w471] -> w469
              stop <- "Save" stop-if-true
              n176 = event shown="[1] \"Section\": Value Change" {
                selector: _ -> [_ _]
                dyn-events: _ -> [_ _]
                timeout: 10 -> [_ _]
                tunnel: w479 -> [w489 w495]
                tunnel: w478 -> [w488 w494]
                tunnel: [w488 w493] -> w472
                tunnel: [w489 w492] -> w473
                tunnel: [_ w491] -> w474
                tunnel: [_ w490] -> w475
                event Timeout {
                  n177 = event-data() -> ()  [unwired: 1 in, 3 out]
                }
                event "Section": Value Change {
                  n178 = event-data() -> ("NewVal"=w491:string)  [unwired: 1 in]
                  n179 = invoke on="Data" class="Tbl (strict)" method="Reinit To Default"() -> ()  [unwired: 3 in, 3 out]
                  n180 = call <vilib>:"Get Key Names.vi"("section"=w491, "error in (no error)"=w494, "refnum"=w495) -> ("error out"=w493:errorcluster, "key names"=w490:string[], "refnum out"=w492:T4)  [unwired: 5 in, 1 out]
                  n181 = property on="Data" class="Tbl (strict)"("Column Headers[]"=w490) -> ()  [unwired: 2 in, 2 out]
                }
              }
              n182 = for {
                tunnel: w475 -> [w486] mode=indexing
                tunnel: w474 -> [w487]
                tunnel: w473 -> [w483]
                tunnel: w472 -> [w482]
                tunnel: [w481] -> w471
                i -> [w485]
                n183 = call-poly <vilib>:"Read Key.vi"("section"=w487, "error in (no error)"=w482, "key"=w486, "refnum"=w483) -> ("error out"=w481:errorcluster, "value"=w484:string)  [unwired: 4 in, 2 out]
                n184 = invoke on="Data" class="Tbl (strict)" method="Set Cell Value"("X Index"=w485, "Y Index"=0, "Value"=w484) -> ()  [unwired: 3 in, 6 out]
              }
            }
          }
          frame #2 {
            w496 = T3."Disabled and Grayed Out" ("Disabled")
            # "Reads all the data in each key and writes it to the file, closes the config file saving the changes and disables the buttons"
            n185 = invoke on="Edit Config" class="Bool" method="Reinit To Default"() -> ()  [unwired: 3 in, 3 out]
            n186 = property on="Data" class="Tbl (strict)"() -> ("Column Headers[]"=w497:string[])  [unwired: 2 in, 2 out]
            n187 = property on="Section" class="CmbBox"() -> ("Value"=w499:string)  [unwired: 2 in, 2 out]
            n188 = for {
              tunnel: w497 -> [w513] mode=indexing
              tunnel: w503 -> [w505]
              tunnel: w499 -> [w508]
              tunnel: [w507] -> w502
              tunnel: [w506] -> w501
              tunnel: w500 -> [w504]
              i -> [w510]
              n189 = property on="Data" class="Tbl (strict)"() -> ("Value"=w512:string[][])  [unwired: 2 in, 2 out]
              n190 = Index Array(array=w512, index (row)=0, index (col)=w510) -> (element=w509:string)
              n191 = call-poly <vilib>:"Write Key.vi"("section"=w508, "error in (no error)"=w504, "value"=w509, "key"=w513, "refnum"=w505) -> ("error out"=w506:errorcluster, "refnum out"=w507:T4)  [unwired: 4 in, 1 out]
            }
            n192 = call <vilib>:"Close Config Data.vi"("error in (no error)"=w501, "refnum"=w502) -> ("error out"=w498:errorcluster)  [unwired: 8 in, 1 out]
            n193 = property on="Save" class="Bool"("DisabledEnum"=w496) -> ()  [unwired: 2 in, 2 out]
            n194 = property on="Section" class="CmbBox"("DisabledEnum"=w496) -> ()  [unwired: 2 in, 2 out]
            n195 = property on="Data" class="Tbl (strict)"("DisabledEnum"=w496) -> ()  [unwired: 2 in, 2 out]
          }
        }
      }
    }
    "Conections" <- w19
    n196 = flat-sequence {
      tunnel: w23 -> [w44]
      tunnel: [w56] -> w21
      frame #0 {
        w48 = errorcluster[] []
        # "Saves the errors in an array while \"retry\" is false, if \"retry\" id true, resets the error array"
        n197 = property on="retry" class="Bool (strict)"() -> ("Value"=w47:bool)  [unwired: 2 in, 2 out]
        n198 = feedback #1(w48) -> (w45:errorcluster[])
        n199 = Select(t=w48, s=w47, f=w45) -> (s? t:f=w49:errorcluster[])
        n200 = case shown="Error" w44 {
          tunnel: w44 -> [_ w54]
          tunnel: [w51 w52] -> w50
          tunnel: w49 -> [w51 w53]
          tunnel: [w51 w52] -> w46
          frame No Error {
          }
          frame Error {
            n201 = Build Array (concatenate)(w53, w54) -> (w52:errorcluster[])
          }
        }
        "Errores" <- w46
        n202 = feedback-in #1(w50) -> ()
      }
      frame #1 {
        # "Sets retry to false and pases the errors to the Handler"
        n203 = property on="Errores" class="Arr (strict)"() -> ("Value"=w56:errorcluster[])  [unwired: 2 in, 2 out]
        n204 = property on="retry" class="Bool (strict)"("Value"=FALSE) -> ()  [unwired: 2 in, 2 out]
      }
    }
    n205 = call "ErrorHandlerSubVI.vi"("Errors"=w21, "queue in"=w24, "Conections In"=w19) -> ("Status"=→"Errors":string[], "queue out"=w22:refnum<queue>)
  }
  n206 = Release Queue(queue=w1, error in (no error)=w2) -> (error out=→"Final Error":errorcluster)  [unwired: 1 in, 2 out]
